vi "MiniCTA.vi"() -> ()   [LabVIEW 2016]
uses:
  controls/DIPBankRadioButton.ctl
  controls/DIPSingleRadioButton.ctl
  <vilib>/printing/EasyPrintingControls.llb/report_type.ctl
  <vilib>/printing/EasyPrintingControls.llb/layout_options.ctl
  <vilib>/printing/EasyPrintingControls.llb/orientation.ctl
  <vilib>/printing/EasyPrintingControls.llb/panel_scaling_for_page.ctl
  <vilib>/printing/EasyPrintingControls.llb/margins.ctl
  <vilib>/printing/EasyPrintingControls.llb/margin_values.ctl
  <vilib>/printing/EasyPrintingControls.llb/measurement_system.ctl
  <vilib>/printing/EasyPrintingControls.llb/printer_options.ctl
  <vilib>/printing/EasyPrintingControls.llb/printing_method.ctl
  <vilib>/printing/EasyPrintingControls.llb/color_or_monochrome.ctl
  <vilib>/printing/EasyPrintingControls.llb/page_header_options.ctl
  <vilib>/printing/EasyPrintingControls.llb/page_headers.ctl
  <vilib>/printing/EasyPrintingControls.llb/page_header_content_options.ctl
  <vilib>/printing/EasyPrintingControls.llb/custom_contents_options.ctl
  <vilib>/printing/EasyPrintingControls.llb/list_which_controls.ctl
  <vilib>/printing/EasyPrinting.llb/Easy Print VI Panel or Documentation (path).vi
  <vilib>/Utility/SMTP/NI_SMTPEmail.lvlib
  <vilib>/Utility/NIReport.llb/NI_ReportGenerationCore.lvlib
panel:
  in  "Tab Control":T1(tab)
  in  "Cable Length (m)":dbl=4.0 min=4.0 max=20.0 step=1.0
  out "SW1":T2
  out "ShortOK":bool
  out "ProbeOK":bool
  in  "Shorted Resistance":dbl min=0.0 max=2.0 step=0.1 format="%.2g"
  in  "Total Resistance":dbl min=0.0 max=100.0 step=0.1 format="%.2g"
  out "SW2":T2
  out "SW3":T2
  out "AllOK?":bool
  out "Cable Resistance":dbl format="%.2g"
  out "Filament\nHot Resistance":dbl format="%.2g"
  in  "alpha":dbl=0.0039
  in  "Overheat":dbl=1.5
  out "Filament\nCold Resistance":dbl format="%.2g"
  out "TargetTotal\nHotResistance":dbl
  out "BridgeSetting":dbl
  out "Rbin":dbl
  out "SW1remainder":dbl
  out "n160":i32
  out "n20":i32
  out "SW2remainder":dbl
  out "n1.4":i32
  out "SW3remainder":dbl
  out "Failed recipients":string[](array[string])
  in  "print?":bool
  in  "Recipients":string[](array[string])=["ttech@cppwind.com"]
  in  "Stop Button":bool
  in  "email?":bool
  in  "mail server":string="post.cppwind.local"
  # "1. Connect probe holder (sting or pigtail type) to 4-10m or 10-20m probe cable; SET DIP  SW1- 3 OR 4 appropriately\n2. Insert shorting probe.\n2. Use CEM DT-5302 (or alternative) Low Resistance Tester on 40 Ohm range to measure shorted holder and cable resistance, and enter displayed value on \"Basic\" tab.\n3. Remove shorting probe and insert hotfilm probe.\n4. Measure total resistance and enter displayed value on \"Basic\" tab.\n5. Set DIP switches as shown- a  dot indicating the switch should be pushed on that side.\n6. Connect the probe cable to the anemometer's \"Probe\" connection.\n7. Power up the bridge by plugging in PSU.\n\nOnly connect probe AFTER switches are set correctly. Power down before unplugging probe."
  # "="
  # "+"
  # "="
  # "X"
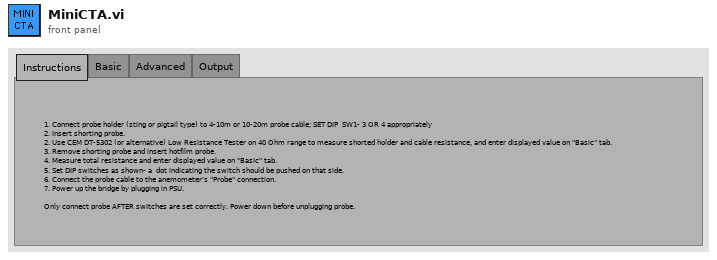
[diagram p1: front panel]
types:
  T1 = enum32{"Instructions", "Basic", "Advanced", "Output"}
  T2 = typedef "DIPBankRadioButton.ctl" = T3[]
  T3 = typedef "DIPSingleRadioButton.ctl" = enum32{"Radio Selection 1", "Radio Selection 2"}
  T4 = cluster{"path":path, "data":string, "binary":bool, "MIME content-type \n(application/octet-stream)":string}
  T5 = typedef "NI_ReportGenerationCore.lvlib/custom_contents_options.ctl" = cluster{"include VI connector and icon":bool, "include VI description":bool, "include front panel":bool, "surround front panel with border":bool, "list of controls options":cluster{"include list of controls":bool, "list which controls?":T6, "include control descriptions?":bool, "include control data types?":bool}, "block diagram options":cluster{"include block diagram":bool, "hidden frames":bool, "ordered (repeat from higher level if nested)":bool}, "include VI hierarchy":bool, "include list of subVIs":bool, "include VI history":bool, "include Express VI configuration information":bool}
  T6 = typedef "NI_ReportGenerationCore.lvlib/list_which_controls.ctl" = u16
  T7 = typedef "NI_ReportGenerationCore.lvlib/layout_options.ctl" = cluster{"orientation (unchanged)":T8, "panel scaling for page (unchanged)":T9, "margins":T10, "printer options":T13, "page header options":T16}
  T8 = typedef "NI_ReportGenerationCore.lvlib/orientation.ctl" = u16
  T9 = typedef "NI_ReportGenerationCore.lvlib/panel_scaling_for_page.ctl" = u16
  T10 = typedef "NI_ReportGenerationCore.lvlib/margins.ctl" = cluster{"override VI margins (false)":bool, "margins (1.00)":T11, "measurement system (default)":T12}
  T11 = typedef "NI_ReportGenerationCore.lvlib/margin_values.ctl" = cluster{"top":dbl, "left":dbl, "right":dbl, "bottom":dbl}
  T12 = typedef "NI_ReportGenerationCore.lvlib/measurement_system.ctl" = u16
  T13 = typedef "NI_ReportGenerationCore.lvlib/printer_options.ctl" = cluster{"destination printer name (current)":string, "printing method (unchanged)":T14, "color or monochrome (unchanged)":T15}
  T14 = typedef "NI_ReportGenerationCore.lvlib/printing_method.ctl" = u16
  T15 = typedef "NI_ReportGenerationCore.lvlib/color_or_monochrome.ctl" = u16
  T16 = typedef "NI_ReportGenerationCore.lvlib/page_header_options.ctl" = cluster{"page headers (unchanged)":T17, "page header content options":T18}
  T17 = typedef "NI_ReportGenerationCore.lvlib/page_headers.ctl" = u16
  T18 = typedef "NI_ReportGenerationCore.lvlib/page_header_content_options.ctl" = cluster{"Include VI Name":bool, "Include VI Path":bool, "Include Last Modification Date":bool, "Include Date Printed":bool, "Include Page Number":bool, "Include VI Icon":bool}
  T19 = typedef "NI_ReportGenerationCore.lvlib/report_type.ctl" = u16
  T20 = cluster{"path":path, "data":string, "binary":bool, "MIME content-type \n(application/octet-stream)":string}[]
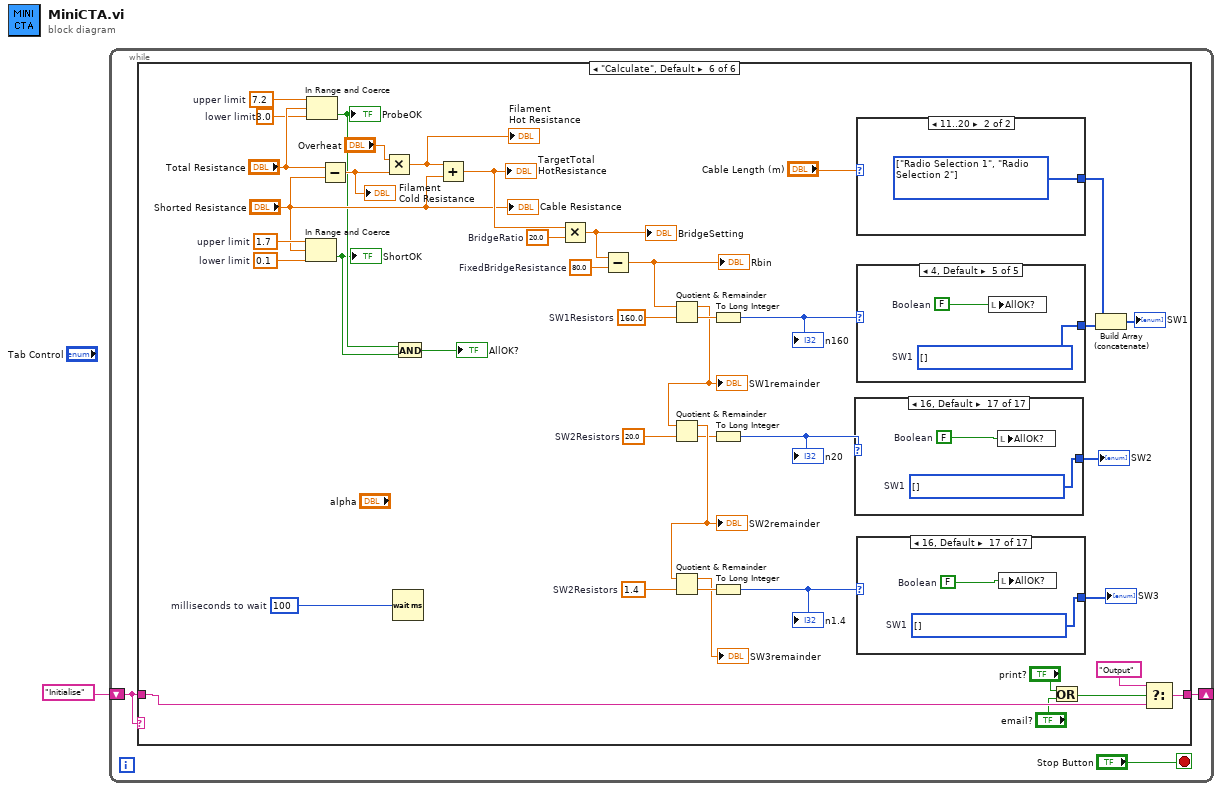
[diagram p0: block diagram]
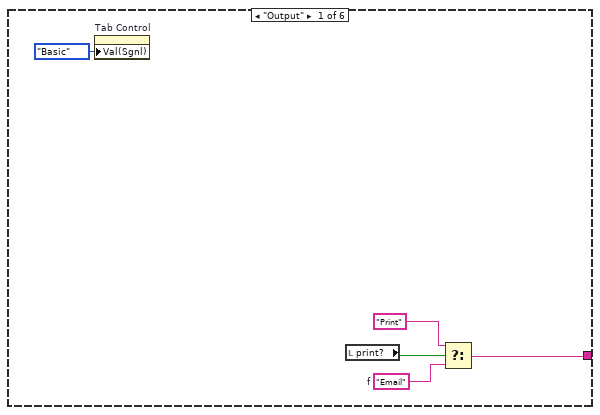
[diagram p2: hidden frame]
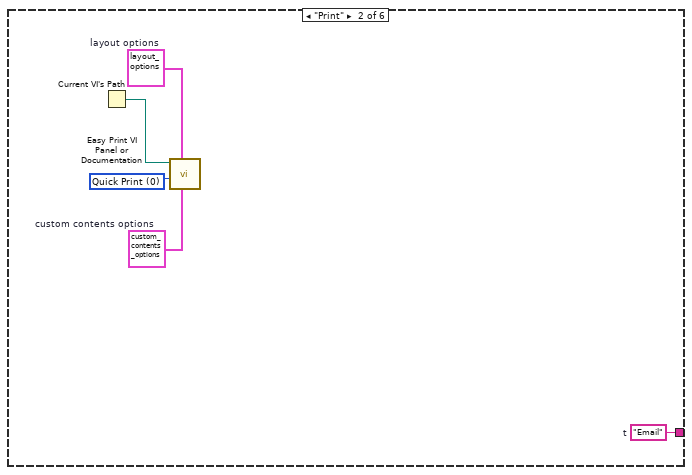
[diagram p3: hidden frame]
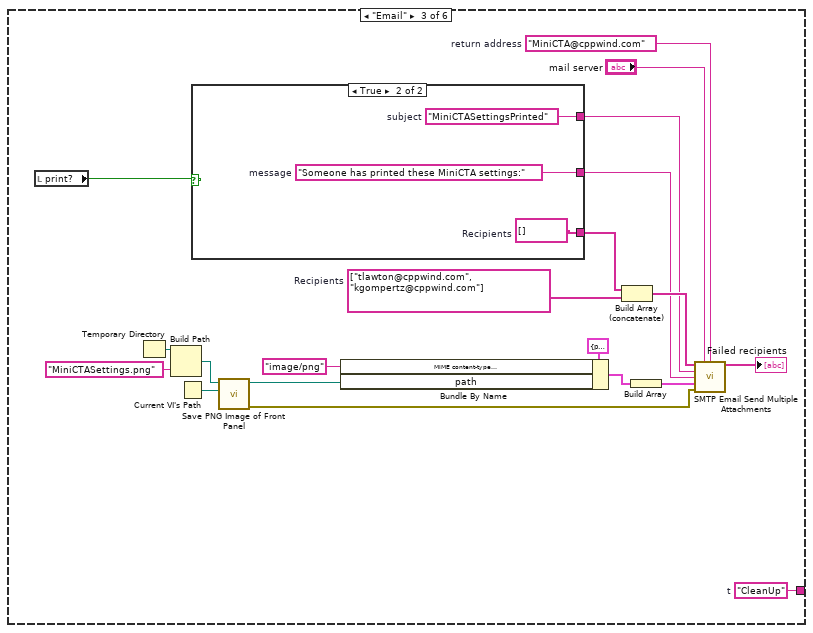
[diagram p4: hidden frame]
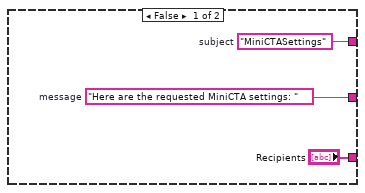
[diagram p5: hidden frame]
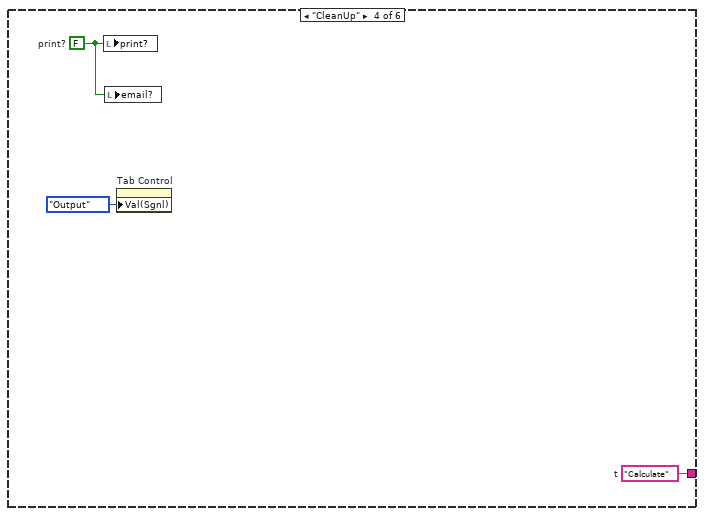
[diagram p6: hidden frame]
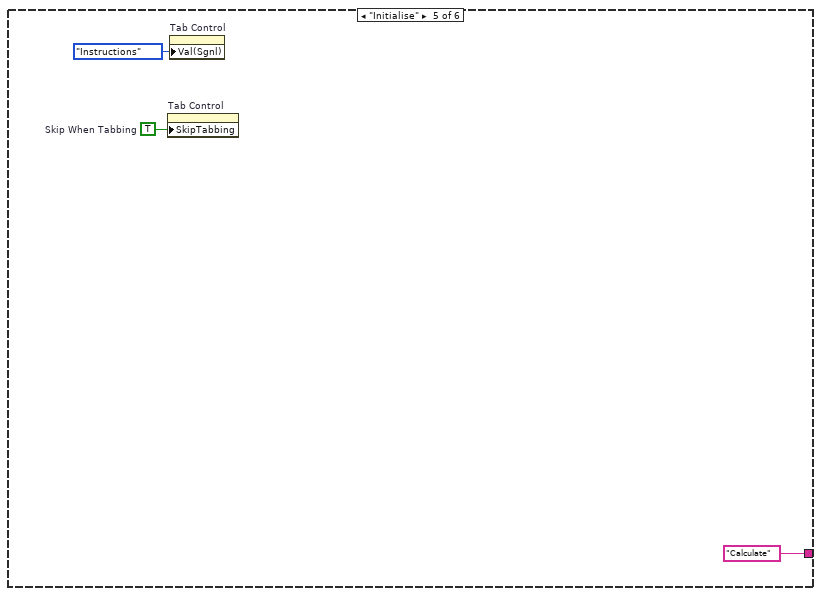
[diagram p7: hidden frame]
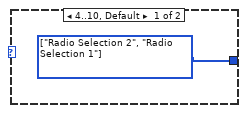
[diagram p8: hidden frame]
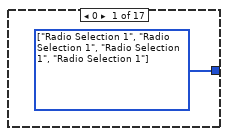
[diagram p9: hidden frame]
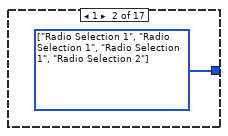
[diagram p10: hidden frame]
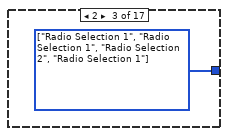
[diagram p11: hidden frame]
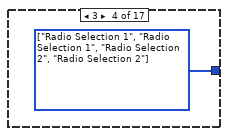
[diagram p12: hidden frame]
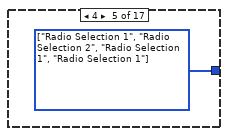
[diagram p13: hidden frame]
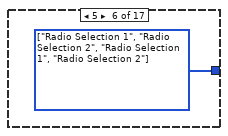
[diagram p14: hidden frame]
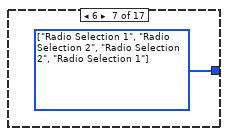
[diagram p15: hidden frame]
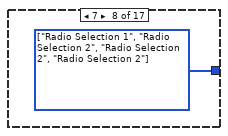
[diagram p16: hidden frame]
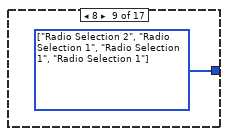
[diagram p17: hidden frame]
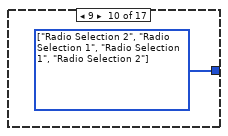
[diagram p18: hidden frame]
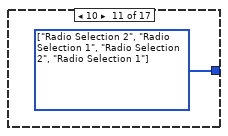
[diagram p19: hidden frame]
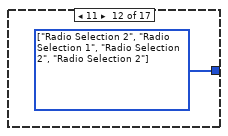
[diagram p20: hidden frame]
diagram:
  n1 = while {
    shift-right: [w2] -> _
    shift-left: "Initialise" -> [w3]
    stop <- "Stop Button" stop-if-true
    n2 = case shown="\"Calculate\", Default" w3 {
      tunnel: w3 -> [_ _ _ _ _ w56]
      tunnel: [w8 w13 w34 w42 "Calculate" w57] -> w2
      frame "Output" {
        w5 = "Email"  # f
        n3 = property on="Tab Control" class="TabCtl (strict)"("Val(Sgnl)"=T1."Basic" ("Value (Signaling)")) -> ()  [unwired: 2 in, 2 out]
        n4 = local read "print?"() -> (w7:bool)
        n5 = Select(t="Print", s=w7, f=w5) -> (s? t:f=w8:string)
      }
      frame "Print" {
        w10 = T5 {"include VI connector and icon"=FALSE, "include VI description"=FALSE, "include front panel"=FALSE, "surround front panel with border"=FALSE, "list of controls options"={"include list of controls"=FALSE, "list which controls?"=0, "include control descriptions?"=FALSE, "include control data types?"=FALSE}, "block diagram options"={"include block diagram"=FALSE, "hidden frames"=FALSE, "ordered (repeat from higher level if nested)"=FALSE}, "include VI hierarchy"=FALSE, "include list of subVIs"=FALSE, "include VI history"=FALSE, "include Express VI configuration information"=FALSE}  # custom contents options
        w11 = T7 {"orientation (unchanged)"=0, "panel scaling for page (unchanged)"=0, "margins"={"override VI margins (false)"=FALSE, "margins (1.00)"={"top"=1.0, "left"=1.0, "right"=1.0, "bottom"=1.0}, "measurement system (default)"=0}, "printer options"={"destination printer name (current)"="", "printing method (unchanged)"=0, "color or monochrome (unchanged)"=0}, "page header options"={"page headers (unchanged)"=1, "page header content options"={"Include VI Name"=FALSE, "Include VI Path"=FALSE, "Include Last Modification Date"=FALSE, "Include Date Printed"=TRUE, "Include Page Number"=FALSE, "Include VI Icon"=FALSE}}}  # layout options
        w12 = T19 0 items=["Quick Print", "Standard Report", "HTML", "Word", "Excel"] ("report type (Quick Print)")
        w13 = "Email"  # t
        n6 = Current VI's Path() -> (path=w14:path)
        n7 = call-poly <vilib>:"Easy Print VI Panel or Documentation.vi"("custom contents options"=w10, "layout options"=w11, "report type (Quick Print)"=w12, "VI path"=w14) -> ()  [unwired: 6 in, 2 out]
      }
      frame "Email" {
        w20 = "MiniCTA@cppwind.com"  # return address
        w23 = string[] ["tlawton@cppwind.com", "kgompertz@cppwind.com"]  # Recipients
        w34 = "CleanUp"  # t
        n8 = local read "print?"() -> (w18:bool)
        n9 = Temporary Directory() -> (w30:path)
        n10 = Build Path(base path=w30, name or relative path="MiniCTASettings.png") -> (appended path=w29:path)
        n11 = Current VI's Path() -> (path=w19:path)
        n12 = case shown="True" w18 {
          tunnel: ["Recipients" w40] -> w21
          tunnel: [w36 w39] -> w17
          tunnel: [w35 w38] -> w15
          frame False {
            w35 = "Here are the requested MiniCTA settings: "  # message
            w36 = "MiniCTASettings"  # subject
          }
          frame True {
            w38 = "Someone has printed these MiniCTA settings:"  # message
            w39 = "MiniCTASettingsPrinted"  # subject
            w40 = string[] []  # Recipients
          }
        }
        n13 = call "Save PNG Image of Front Panel.vi"("VI Path"=w19, "File Path In"=w29) -> ("error out"=w24:errorcluster, "File Path Out"=w31:path)  [unwired: 8 in]
        n14 = Bundle By Name(cluster=T4 {"path"=path "", "data"="", "binary"=TRUE, "MIME content-type \n(application/octet-stream)"="application/octet-stream"}, "MIME content-type \n(application/octet-stream)"="image/png" ("MIME content-type \n(application/octet-stream)"), "path"=w31) -> (w27:T4)
        n15 = Build Array (concatenate)(w21, w23) -> (w22:string[])
        n16 = Build Array(w27) -> (w26:T20)
        n17 = call <vilib>:"SMTP Email Send Multiple Attachments.vi"("recipients"=w22, "mail server"="mail server", "return address"=w20, "subject ([No Subject])"=w17, "message"=w15, "attachments"=w26, "error in (no error)"=w24) -> ("invalid recipients"=→"Failed recipients":string[])  [unwired: 7 in, 1 out]
      }
      frame "CleanUp" {
        w42 = "Calculate"  # t
        w43 = FALSE  # print?
        n18 = local write "print?"(w43) -> ()
        n19 = local write "email?"(w43) -> ()
        n20 = property on="Tab Control" class="TabCtl (strict)"("Val(Sgnl)"=T1."Output" ("Value (Signaling)")) -> ()  [unwired: 2 in, 2 out]
      }
      frame "Initialise" {
        w44 = TRUE  # Skip When Tabbing
        n21 = property on="Tab Control" class="TabCtl (strict)"("SkipTabbing"=w44) -> ()  [unwired: 2 in, 2 out]
        n22 = property on="Tab Control" class="TabCtl (strict)"("Val(Sgnl)"=T1."Instructions" ("Value (Signaling)")) -> ()  [unwired: 2 in, 2 out]
      }
      frame "Calculate", Default {
        w61 = 7.2  # upper limit
        w62 = 3.0  # lower limit
        w64 = 0.1  # lower limit
        w65 = 1.7  # upper limit
        w66 = u32 100  # milliseconds to wait
        w75 = 1.4  # SW2Resistors
        w78 = 20.0  # SW2Resistors
        w81 = 160.0  # SW1Resistors
        w83 = 80.0  # FixedBridgeResistance
        w85 = 20.0  # BridgeRatio
        n23 = In Range and Coerce(upper limit=w65, x="Shorted Resistance", lower limit=w64) -> (In Range?=w48:bool)  [unwired: 1 out]
        "ShortOK" <- w48
        n24 = In Range and Coerce(upper limit=w61, x="Total Resistance", lower limit=w62) -> (In Range?=w49:bool)  [unwired: 1 out]
        "ProbeOK" <- w49
        n25 = Subtract(x="Total Resistance", y="Shorted Resistance") -> (x-y=w88:dbl)
        "Filament\nCold Resistance" <- w88
        n26 = Multiply(x="Overheat", y=w88) -> (x*y=w51:dbl)
        "Filament\nHot Resistance" <- w51
        n27 = Wait (ms)(milliseconds to wait=w66) -> ()  [unwired: 1 out]
        n28 = And(x=w49, y=w48) -> (x .and. y?=→"AllOK?":bool)
        n29 = Add(x=w51, y="Shorted Resistance") -> (x+y=w86:dbl)
        "TargetTotal\nHotResistance" <- w86
        n30 = Multiply(x=w86, y=w85) -> (x*y=w84:dbl)
        "BridgeSetting" <- w84
        n31 = Subtract(x=w84, y=w83) -> (x-y=w82:dbl)
        "Rbin" <- w82
        n32 = Quotient & Remainder(x=w82, y=w81) -> (x-y*floor(x/y)=w77:dbl, floor(x/y)=w80:dbl)
        "SW1remainder" <- w77
        n33 = Quotient & Remainder(x=w77, y=w78) -> (x-y*floor(x/y)=w74:dbl, floor(x/y)=w71:dbl)
        "SW2remainder" <- w74
        n34 = Quotient & Remainder(x=w74, y=w75) -> (x-y*floor(x/y)=→"SW3remainder":dbl, floor(x/y)=w69:dbl)
        n35 = To Long Integer(number=w80) -> (32bit integer=w72:i32)
        "n160" <- w72
        n36 = To Long Integer(number=w71) -> (32bit integer=w70:i32)
        "n20" <- w70
        n37 = To Long Integer(number=w69) -> (32bit integer=w68:i32)
        "n1.4" <- w68
        n38 = case shown="16, Default" w70 {
          tunnel: [w109 w110 w111 w112 w113 w114 w115 w116 w117 w118 w119 w120 w121 w122 w123 w124 w126] -> w76
          frame 0 {
            w109 = T2 [enum."Radio Selection 1", enum."Radio Selection 1", enum."Radio Selection 1", enum."Radio Selection 1"] items=["Radio Selection 1", "Radio Selection 2"] ("SW1")
          }
          frame 1 {
            w110 = T2 [enum."Radio Selection 1", enum."Radio Selection 1", enum."Radio Selection 1", enum."Radio Selection 2"] items=["Radio Selection 1", "Radio Selection 2"] ("SW1")
          }
          frame 2 {
            w111 = T2 [enum."Radio Selection 1", enum."Radio Selection 1", enum."Radio Selection 2", enum."Radio Selection 1"] items=["Radio Selection 1", "Radio Selection 2"] ("SW1")
          }
          frame 3 {
            w112 = T2 [enum."Radio Selection 1", enum."Radio Selection 1", enum."Radio Selection 2", enum."Radio Selection 2"] items=["Radio Selection 1", "Radio Selection 2"] ("SW1")
          }
          frame 4 {
            w113 = T2 [enum."Radio Selection 1", enum."Radio Selection 2", enum."Radio Selection 1", enum."Radio Selection 1"] items=["Radio Selection 1", "Radio Selection 2"] ("SW1")
          }
          frame 5 {
            w114 = T2 [enum."Radio Selection 1", enum."Radio Selection 2", enum."Radio Selection 1", enum."Radio Selection 2"] items=["Radio Selection 1", "Radio Selection 2"] ("SW1")
          }
          frame 6 {
            w115 = T2 [enum."Radio Selection 1", enum."Radio Selection 2", enum."Radio Selection 2", enum."Radio Selection 1"] items=["Radio Selection 1", "Radio Selection 2"] ("SW1")
          }
          frame 7 {
            w116 = T2 [enum."Radio Selection 1", enum."Radio Selection 2", enum."Radio Selection 2", enum."Radio Selection 2"] items=["Radio Selection 1", "Radio Selection 2"] ("SW1")
          }
          frame 8 {
            w117 = T2 [enum."Radio Selection 2", enum."Radio Selection 1", enum."Radio Selection 1", enum."Radio Selection 1"] items=["Radio Selection 1", "Radio Selection 2"] ("SW1")
          }
          frame 9 {
            w118 = T2 [enum."Radio Selection 2", enum."Radio Selection 1", enum."Radio Selection 1", enum."Radio Selection 2"] items=["Radio Selection 1", "Radio Selection 2"] ("SW1")
          }
          frame 10 {
            w119 = T2 [enum."Radio Selection 2", enum."Radio Selection 1", enum."Radio Selection 2", enum."Radio Selection 1"] items=["Radio Selection 1", "Radio Selection 2"] ("SW1")
          }
          frame 11 {
            w120 = T2 [enum."Radio Selection 2", enum."Radio Selection 1", enum."Radio Selection 2", enum."Radio Selection 2"] items=["Radio Selection 1", "Radio Selection 2"] ("SW1")
          }
          frame 12 {
            w121 = T2 [enum."Radio Selection 2", enum."Radio Selection 2", enum."Radio Selection 1", enum."Radio Selection 1"] items=["Radio Selection 1", "Radio Selection 2"] ("SW1")
          }
          frame 13 {
            w122 = T2 [enum."Radio Selection 2", enum."Radio Selection 2", enum."Radio Selection 1", enum."Radio Selection 2"] items=["Radio Selection 1", "Radio Selection 2"] ("SW1")
          }
          frame 14 {
            w123 = T2 [enum."Radio Selection 2", enum."Radio Selection 2", enum."Radio Selection 2", enum."Radio Selection 1"] items=["Radio Selection 1", "Radio Selection 2"] ("SW1")
          }
          frame 15 {
            w124 = T2 [enum."Radio Selection 2", enum."Radio Selection 2", enum."Radio Selection 2", enum."Radio Selection 2"] items=["Radio Selection 1", "Radio Selection 2"] ("SW1")
          }
          frame 16, Default {
            w125 = FALSE  # Boolean
            w126 = T2 [] items=["Radio Selection 1", "Radio Selection 2"]  # SW1
            n39 = local write "AllOK?"(w125) -> ()
          }
        }
        "SW2" <- w76
        n40 = case shown="11..20" "Cable Length (m)" {
          tunnel: [w89 w90] -> w58
          frame 4..10, Default {
            w89 = T2 [enum."Radio Selection 2", enum."Radio Selection 1"] items=["Radio Selection 1", "Radio Selection 2"] ("SW1")
          }
          frame 11..20 {
            w90 = T2 [enum."Radio Selection 1", enum."Radio Selection 2"] items=["Radio Selection 1", "Radio Selection 2"] ("SW1")
          }
        }
        n41 = case shown="4, Default" w72 {
          tunnel: [w127 w128 w129 w130 w132] -> w79
          frame 0 {
            w127 = T2 [enum."Radio Selection 1", enum."Radio Selection 1"] items=["Radio Selection 1", "Radio Selection 2"] ("SW1")
          }
          frame 1 {
            w128 = T2 [enum."Radio Selection 1", enum."Radio Selection 2"] items=["Radio Selection 1", "Radio Selection 2"] ("SW1")
          }
          frame 2 {
            w129 = T2 [enum."Radio Selection 2", enum."Radio Selection 2"] items=["Radio Selection 1", "Radio Selection 2"] ("SW1")
          }
          frame 3 {
            w130 = T2 [enum."Radio Selection 1", enum."Radio Selection 1"] items=["Radio Selection 1", "Radio Selection 2"] ("SW1")
          }
          frame 4, Default {
            w131 = FALSE  # Boolean
            w132 = T2 [] items=["Radio Selection 1", "Radio Selection 2"]  # SW1
            n42 = local write "AllOK?"(w131) -> ()
          }
        }
        n43 = case shown="16, Default" w68 {
          tunnel: [w91 w92 w93 w94 w95 w96 w97 w98 w99 w100 w101 w102 w103 w104 w105 w106 w108] -> w73
          frame 0 {
            w91 = T2 [enum."Radio Selection 1", enum."Radio Selection 1", enum."Radio Selection 1", enum."Radio Selection 1"] items=["Radio Selection 1", "Radio Selection 2"] ("SW1")
          }
          frame 1 {
            w92 = T2 [enum."Radio Selection 1", enum."Radio Selection 1", enum."Radio Selection 1", enum."Radio Selection 2"] items=["Radio Selection 1", "Radio Selection 2"] ("SW1")
          }
          frame 2 {
            w93 = T2 [enum."Radio Selection 1", enum."Radio Selection 1", enum."Radio Selection 2", enum."Radio Selection 1"] items=["Radio Selection 1", "Radio Selection 2"] ("SW1")
          }
          frame 3 {
            w94 = T2 [enum."Radio Selection 1", enum."Radio Selection 1", enum."Radio Selection 2", enum."Radio Selection 2"] items=["Radio Selection 1", "Radio Selection 2"] ("SW1")
          }
          frame 4 {
            w95 = T2 [enum."Radio Selection 1", enum."Radio Selection 2", enum."Radio Selection 1", enum."Radio Selection 1"] items=["Radio Selection 1", "Radio Selection 2"] ("SW1")
          }
          frame 5 {
            w96 = T2 [enum."Radio Selection 1", enum."Radio Selection 2", enum."Radio Selection 1", enum."Radio Selection 2"] items=["Radio Selection 1", "Radio Selection 2"] ("SW1")
          }
          frame 6 {
            w97 = T2 [enum."Radio Selection 1", enum."Radio Selection 2", enum."Radio Selection 2", enum."Radio Selection 1"] items=["Radio Selection 1", "Radio Selection 2"] ("SW1")
          }
          frame 7 {
            w98 = T2 [enum."Radio Selection 1", enum."Radio Selection 2", enum."Radio Selection 2", enum."Radio Selection 2"] items=["Radio Selection 1", "Radio Selection 2"] ("SW1")
          }
          frame 8 {
            w99 = T2 [enum."Radio Selection 2", enum."Radio Selection 1", enum."Radio Selection 1", enum."Radio Selection 1"] items=["Radio Selection 1", "Radio Selection 2"] ("SW1")
          }
          frame 9 {
            w100 = T2 [enum."Radio Selection 2", enum."Radio Selection 1", enum."Radio Selection 1", enum."Radio Selection 2"] items=["Radio Selection 1", "Radio Selection 2"] ("SW1")
          }
          frame 10 {
            w101 = T2 [enum."Radio Selection 2", enum."Radio Selection 1", enum."Radio Selection 2", enum."Radio Selection 1"] items=["Radio Selection 1", "Radio Selection 2"] ("SW1")
          }
          frame 11 {
            w102 = T2 [enum."Radio Selection 2", enum."Radio Selection 1", enum."Radio Selection 2", enum."Radio Selection 2"] items=["Radio Selection 1", "Radio Selection 2"] ("SW1")
          }
          frame 12 {
            w103 = T2 [enum."Radio Selection 2", enum."Radio Selection 2", enum."Radio Selection 1", enum."Radio Selection 1"] items=["Radio Selection 1", "Radio Selection 2"] ("SW1")
          }
          frame 13 {
            w104 = T2 [enum."Radio Selection 2", enum."Radio Selection 2", enum."Radio Selection 1", enum."Radio Selection 2"] items=["Radio Selection 1", "Radio Selection 2"] ("SW1")
          }
          frame 14 {
            w105 = T2 [enum."Radio Selection 2", enum."Radio Selection 2", enum."Radio Selection 2", enum."Radio Selection 1"] items=["Radio Selection 1", "Radio Selection 2"] ("SW1")
          }
          frame 15 {
            w106 = T2 [enum."Radio Selection 2", enum."Radio Selection 2", enum."Radio Selection 2", enum."Radio Selection 2"] items=["Radio Selection 1", "Radio Selection 2"] ("SW1")
          }
          frame 16, Default {
            w107 = FALSE  # Boolean
            w108 = T2 [] items=["Radio Selection 1", "Radio Selection 2"]  # SW1
            n44 = local write "AllOK?"(w107) -> ()
          }
        }
        "SW3" <- w73
        n45 = Or(x="print?", y="email?") -> (x .or. y?=w53:bool)
        n46 = Build Array (concatenate)(w58, w79) -> (→"SW1":T2)
        n47 = Select(t="Output", s=w53, f=w56) -> (s? t:f=w57:string)
        "Cable Resistance" <- "Shorted Resistance"
      }
    }
  }
